vi "readCSV_.vi"(8 "error in (no error)":errorcluster, 10 "file path (use dialog)":path=path "C:/Users/RoboIme/git/sslview/Util/Farias2.csv", 11 "Utilities in":refnum<class "Utilities.lvclass">) -> (0 "error out":errorcluster, 2 "array":dbl[][](array[numeric]), 3 "Utilities out":refnum<class "Utilities.lvclass">)   [LabVIEW 2023, in "Utilities.lvclass"]
uses:
  Utilities.lvclass
panel:
  out "refnum out":refnum<file>
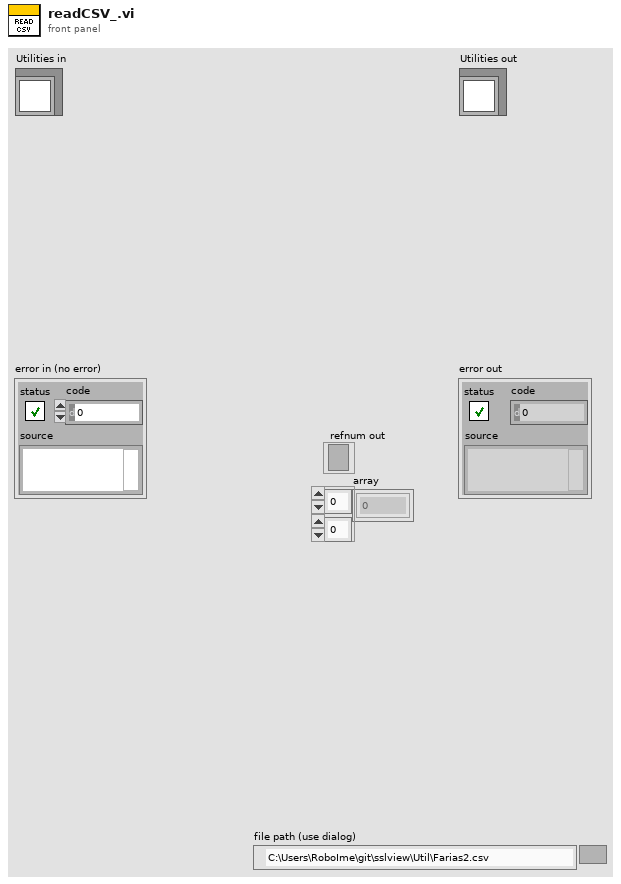
[diagram p1: front panel]
types:
  T1 = enum16{"open", "replace", "create", "open or create", "replace or create", "replace or create with confirmation"}
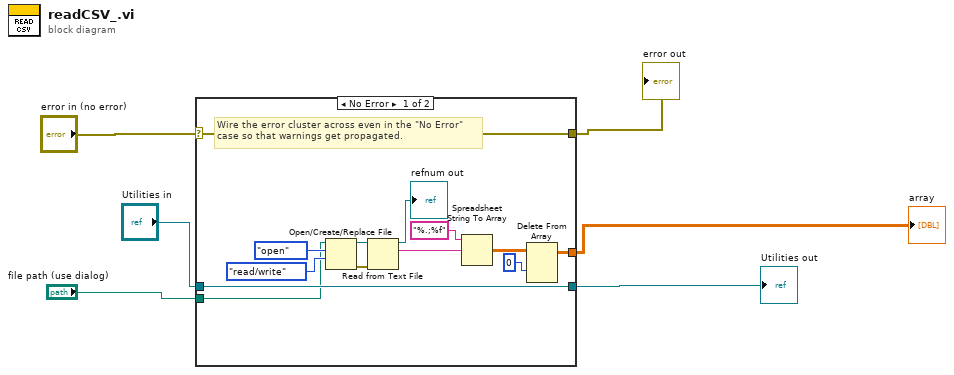
[diagram p0: block diagram]
diagram:
  n1 = case shown="No Error" "error in (no error)" {
    selector: "error in (no error)" -> [w18 w21]
    tunnel: [w18 w21] -> w5
    tunnel: [w19 w20] -> w3
    tunnel: "Utilities in" -> [w19 w20]
    tunnel: "file path (use dialog)" -> [w15 _]
    tunnel: [w8 _] -> w1
    frame No Error {
      # "Wire the error cluster across even in the \"No Error\"\ncase so that warnings get propagated."
      n2 = Open/Create/Replace File(file path (use dialog)=w15, operation (0:open)=T1."open", access (0:read/write)=enum16{"read/write", "read-only", "write-only"}."read/write") -> (refnum out=w14:refnum<file>, error out=w7:errorcluster)  [unwired: 3 in, 1 out]
      n3 = Read from Text File(file (use dialog)=w14, error in=w7) -> (refnum out=→"refnum out":refnum<file>, text=w12:string)  [unwired: 2 in, 2 out]
      n4 = Spreadsheet String To Array(format string="%.;%f", spreadsheet string=w12) -> (array=w10:dbl[][])  [unwired: 2 in]
      n5 = Delete From Array(array=w10, index (row)=0) -> (array with subset deleted=w8:dbl[][])  [unwired: 2 in, 1 out]
    }
    frame Error {
    }
  }
  "error out" <- w5
  "Utilities out" <- w3
  "array" <- w1
